vi "MQTT-subscriber.vi"() -> ()   [LabVIEW 2020]
uses:
  <vilib>/LabVIEW Open Source Project/MQTT Client/Client class/Client.lvclass/Client.ctl
  <vilib>/LabVIEW Open Source Project/MQTT Connection/MQTT_Base/Base Class/MQTT_Base.lvclass/MQTT_Base.ctl
  <vilib>/LabVIEW Open Source Project/Connection/Connection.TCP/Connection.TCP.lvclass
  C:/Program Files (x86)/National Instruments/LabVIEW 2020/vi.lib/LabVIEW Open Source Project/Connection/Connection/Connection.lvclass
  <vilib>/LabVIEW Open Source Project/MQTT Client/Client class/Client.lvclass
  C:/Program Files (x86)/National Instruments/LabVIEW 2020/vi.lib/LabVIEW Open Source Project/MQTT Connection/MQTT_Base/Base Class/MQTT_Base.lvclass
  <vilib>/LabVIEW Open Source Project/MQTT Control Packets/Control Packets/PUBLISH/PUBLISH.lvclass
  <vilib>/LabVIEW Open Source Project/MQTT Connection/MQTT_Base/Base Class/MQTT_Base.lvclass
  <vilib>/LabVIEW Open Source Project/Connection/Connection.LocalQueue/Connection.LocalQueue.lvclass
  <vilib>/LabVIEW Open Source Project/Connection/Connection/Connection.lvclass
panel:
  out "Payload":variant
  out "Unsuback":bool
  out "Suback":bool
  in  "Subscribe":bool
  in  "Connection":bool
  in  "Stop Client":bool
  out "last error":errorcluster
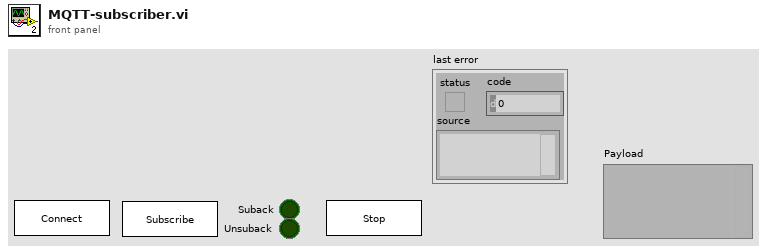
[diagram p1: front panel]
types:
  T1 = typedef "MQTT Client.lvlib/Client.lvclass/Public Events -- cluster.ctl" = cluster{"Connection Status":refnum<user-event>, "Connected":refnum<user-event>, "Application Message":refnum<user-event>}
  T2 = typedef "MQTT Base.lvlib/MQTT_Base.lvclass/Public Events -- cluster.ctl" = cluster{"Stop Event":refnum<user-event>, "Error Event":refnum<user-event>, "Inbound Message":refnum<user-event>}
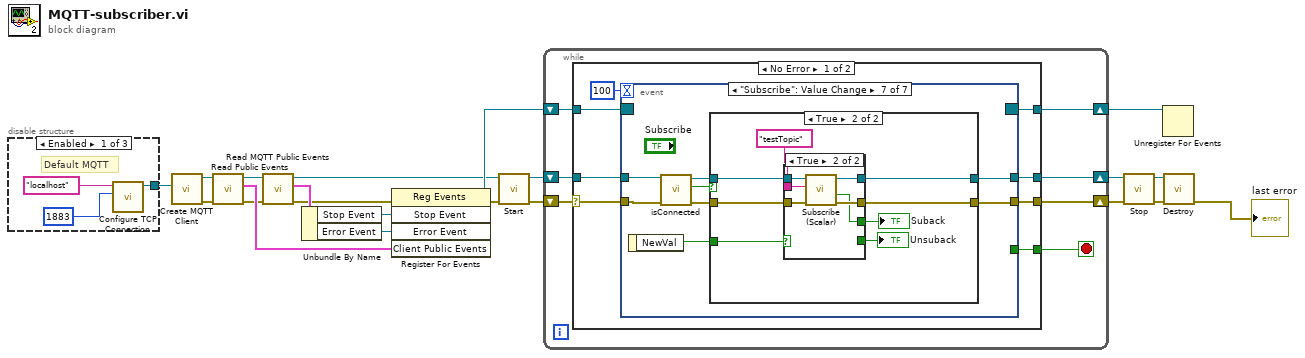
[diagram p0: block diagram]
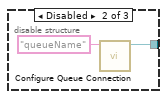
[diagram p2: hidden frame]
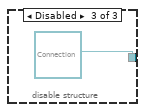
[diagram p3: hidden frame]
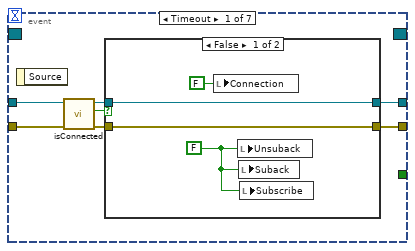
[diagram p4: hidden frame]
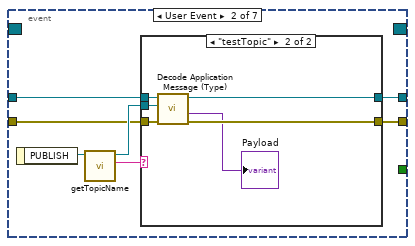
[diagram p6: hidden frame]
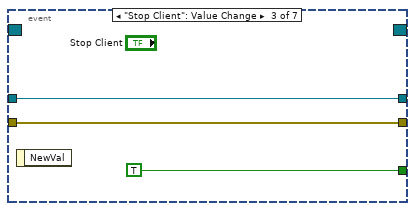
[diagram p8: hidden frame]
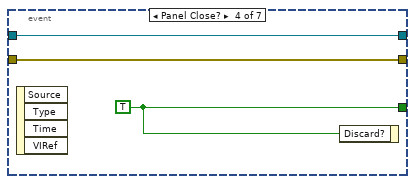
[diagram p9: hidden frame]
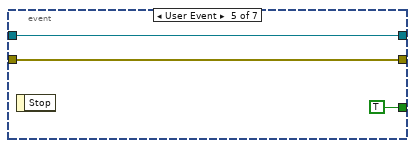
[diagram p10: hidden frame]
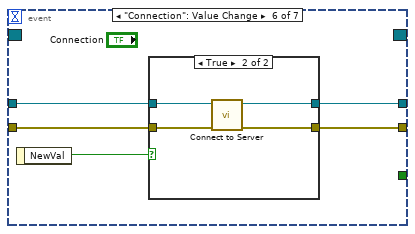
[diagram p11: hidden frame]
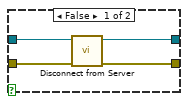
[diagram p12: hidden frame]
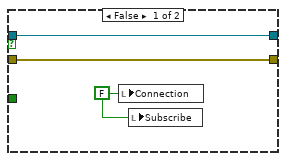
[diagram p13: hidden frame]
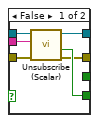
[diagram p14: hidden frame]
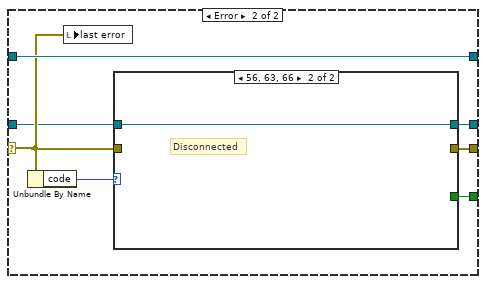
[diagram p15: hidden frame]
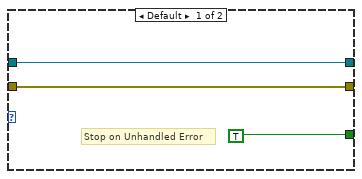
[diagram p16: hidden frame]
diagram:
  n1 = disable-structure shown="Enabled" {
    disable-tunnel: [w23 w26 refnum<class "Connection.lvclass"> refnum ("Connection Configuration")] -> w21
    frame Enabled {
      # "Default MQTT"
      n2 = call <vilib>:"Configure TCP Connection.vi"("remote port (80)"=u16 1883, "address (localhost)"="localhost") -> ("Connection.TCP"=w23:refnum<class "Connection.TCP.lvclass">)  [unwired: 8 in, 1 out]
    }
    frame Disabled {
      n3 = call <vilib>:"Configure Queue Connection.vi"("Queue Name"="queueName") -> ("Connection.LocalQueue"=w26:refnum<class "Connection.LocalQueue.lvclass">)  [unwired: 9 in, 1 out]
    }
    frame Disabled {
    }
  }
  n4 = call <vilib>:"Create MQTT Client.vi"("Connection Configuration"=w21) -> ("error out"=w3:errorcluster, "Client out"=w1:refnum<class "Client.lvclass">)  [unwired: 9 in]
  n5 = call <vilib>:"Read Public Events.vi"("error in (no error)"=w3, "Client in"=w1) -> ("error out"=w4:errorcluster, "Client Public Events"=w6:T1, "Client out"=w2:refnum<class "Client.lvclass">)  [unwired: 7 in]
  n6 = call <vilib>:"Read MQTT Public Events.vi"("error in (no error)"=w4, "MQTT_Base in"=w2) -> ("error out"=w5:errorcluster, "MQTT Public Events"=w13:T2, "MQTT_Base out"=w8:refnum<class "Client.lvclass">)  [unwired: 7 in]
  n7 = Unbundle By Name(w13) -> ("Stop Event"=w11:refnum<user-event>, "Error Event"=w12:refnum<user-event>)
  n8 = register-events(error in=w5, w11, w12, w6) -> (reference out=w9:refnum<event-registration>, error out=w7:errorcluster)  [unwired: 1 in]
  n9 = call <vilib>:"Start.vi"("error in (no error)"=w7, "MQTT_Base in"=w8) -> ("error out"=w19:errorcluster, "MQTT_Base out"=w18:refnum<class "Client.lvclass">)  [unwired: 7 in, 1 out]
  n10 = while {
    shift-right: [w33] -> w10
    shift-left: w9 -> [w34]
    shift-right: [w30] -> w15
    shift-left: w18 -> [w31]
    shift-right: [w32] -> w17
    shift-left: w19 -> [w28]
    stop <- w29 stop-if-true
    n11 = case shown="No Error" w28 {
      selector: w28 -> [w35 w127]
      tunnel: w34 -> [w42 w130]
      tunnel: [w41 w130] -> w33
      tunnel: [w40 w125] -> w32
      tunnel: w31 -> [w38 w126]
      tunnel: [w37 w129] -> w30
      tunnel: [w36 w124] -> w29
      frame No Error {
        n12 = event shown="[6] \"Subscribe\": Value Change" {
          selector: w42 -> [_ _ _ _ _ _ _]
          dyn-events: [_ _ _ _ _ _ _] -> w41
          timeout: 100 -> [_ _ _ _ _ _ _]
          tunnel: w35 -> [w45 w59 w72 w74 w79 w80 w98]
          tunnel: [w48 w56 w72 w74 w79 w81 w99] -> w40
          tunnel: [_ _ TRUE w76 TRUE _ _] -> w36
          tunnel: w38 -> [w47 w60 w73 w75 w77 w84 w97]
          tunnel: [w49 w58 w73 w75 w77 w82 w100] -> w37
          event Timeout {
            n13 = event-data() -> ()  [unwired: 1 in, 1 out]
            n14 = call <vilib>:"isConnected.vi"("error in (no error)"=w45, "Client in"=w47) -> ("error out"=w44:errorcluster, "connected"=w43:bool, "Client out"=w46:refnum<class "Client.lvclass">)  [unwired: 7 in]
            n15 = case shown="False" w43 {
              tunnel: [w53 w55] -> w49
              tunnel: [w52 w54] -> w48
              tunnel: w46 -> [w53 w55]
              tunnel: w44 -> [w52 w54]
              frame False {
                w51 = FALSE
                n16 = local write "Connection"(FALSE ("Connection")) -> ()
                n17 = local write "Unsuback"(w51) -> ()
                n18 = local write "Suback"(w51) -> ()
                n19 = local write "Subscribe"(w51) -> ()
              }
              frame True {
              }
            }
          }
          event User Event {
            n20 = event-data() -> ("PUBLISH"=w62:refnum<class "PUBLISH.lvclass">)  [unwired: 1 in]
            n21 = call <vilib>:"getTopicName.vi"("PUBLISH in"=w62) -> ("Topic"=w57:string, "PUBLISH out"=w61:refnum<class "PUBLISH.lvclass">)  [unwired: 8 in, 1 out]
            n22 = case shown="\"testTopic\"" w57 {
              tunnel: w61 -> [_ w67]
              tunnel: w60 -> [w64 w70]
              tunnel: w59 -> [w63 w68]
              tunnel: [w64 w69] -> w58
              tunnel: [w63 w66] -> w56
              frame Default {
              }
              frame "testTopic" {
                n23 = call <vilib>:"Decode Application Message (Type).vi"("error in (no error)"=w68, "PUBLISH"=w67, "Client in"=w70) -> ("error out"=w66:errorcluster, "Payload"=→"Payload":variant, "Client out"=w69:refnum<class "Client.lvclass">)  [unwired: 5 in, 1 out]
              }
            }
          }
          event "Stop Client": Value Change {
            n24 = event-data() -> ()  [unwired: 1 in, 1 out]
          }
          event Panel Close? {
            w76 = TRUE
            n25 = event-data() -> ()  [unwired: 1 in, 4 out]
            n26 = event-data("Discard?"=w76) -> ()  [unwired: 1 in, 1 out]
          }
          event User Event {
            n27 = event-data() -> ()  [unwired: 1 in, 1 out]
          }
          event "Connection": Value Change {
            n28 = event-data() -> ("NewVal"=w83:bool)  [unwired: 1 in]
            n29 = case shown="True" w83 {
              tunnel: w84 -> [w88 w92]
              tunnel: [w87 w89] -> w82
              tunnel: [w86 w90] -> w81
              tunnel: w80 -> [w85 w91]
              frame False {
                n30 = call <vilib>:"Disconnect from Server.vi"("error in (no error)"=w85, "Client in"=w88) -> ("error out"=w86:errorcluster, "Client out"=w87:refnum<class "Client.lvclass">)  [unwired: 7 in, 1 out]
              }
              frame True {
                n31 = call <vilib>:"Connect to Server.vi"("error in (no error)"=w91, "Client in"=w92) -> ("error out"=w90:errorcluster, "Client out"=w89:refnum<class "Client.lvclass">)  [unwired: 6 in, 2 out]
              }
            }
          }
          event "Subscribe": Value Change {
            n32 = event-data() -> ("NewVal"=w93:bool)  [unwired: 1 in]
            n33 = call <vilib>:"isConnected.vi"("error in (no error)"=w98, "Client in"=w97) -> ("error out"=w95:errorcluster, "connected"=w94:bool, "Client out"=w96:refnum<class "Client.lvclass">)  [unwired: 7 in]
            n34 = case shown="True" w94 {
              tunnel: [w103 w111] -> w100
              tunnel: [w102 w110] -> w99
              tunnel: w96 -> [w103 w109]
              tunnel: w95 -> [w102 w108]
              tunnel: w93 -> [_ w106]
              frame False {
                w101 = FALSE ("Connection")
                n35 = local write "Connection"(w101) -> ()
                n36 = local write "Subscribe"(w101) -> ()
              }
              frame True {
                n37 = case shown="True" w106 {
                  tunnel: [w112 w120] -> w111
                  tunnel: [w113 w119] -> w110
                  tunnel: w109 -> [w117 w123]
                  tunnel: w108 -> [w116 w122]
                  tunnel: "testTopic" ("Topic Name (empty: Payload name)") -> [w115 w121]
                  tunnel: [_ w118] -> w105
                  tunnel: [w114 _] -> w104
                  frame False {
                    n38 = call <vilib>:"Unsubscribe (Scalar).vi"("error in (no error)"=w116, "Topic Filter"=w115, "Client in"=w117) -> ("error out"=w113:errorcluster, "Ack"=w114:bool, "Client out"=w112:refnum<class "Client.lvclass">)  [unwired: 6 in]
                  }
                  frame True {
                    n39 = call <vilib>:"Subscribe (Scalar).vi"("error in (no error)"=w122, "Topic Filter"=w121, "Client in"=w123) -> ("error out"=w119:errorcluster, "Ack"=w118:bool, "Client out"=w120:refnum<class "Client.lvclass">)  [unwired: 6 in]
                  }
                }
                "Unsuback" <- w104
                "Suback" <- w105
              }
            }
          }
        }
      }
      frame Error {
        n40 = Unbundle By Name(w127) -> ("code"=w128:i32)
        n41 = local write "last error"(w127) -> ()
        n42 = case shown="56, 63, 66" w128 {
          tunnel: w126 -> [w133 w134]
          tunnel: [w133 w134] -> w129
          tunnel: w127 -> [w132 _]
          tunnel: [w132 _] -> w125
          tunnel: [TRUE _] -> w124
          frame Default {
            # "Stop on Unhandled Error"
          }
          frame 56, 63, 66 {
            # "Disconnected"
          }
        }
      }
    }
  }
  n43 = call <vilib>:"Stop.vi"("error in (no error)"=w17, "MQTT_Base in"=w15) -> ("error out"=w16:errorcluster, "MQTT_Base out"=w14:refnum<class "Client.lvclass">)  [unwired: 7 in, 1 out]
  n44 = Unregister For Events(event registration refnum=w10) -> ()  [unwired: 1 in, 1 out]
  n45 = call <vilib>:"Destroy.vi"("error in (no error)"=w16, "MQTT_Base in"=w14) -> ("error out"=→"last error":errorcluster)  [unwired: 8 in, 1 out]
